vi "5492_AutonomousTurn.vi"(8 "error in (no error)":errorcluster, 9 "RobotDriveDevRef":T1={"DevStatus"={"status"=FALSE, "code"=0, "source"=""}, "Motors[]"=[], "Square Inputs"=FALSE, "Max Output"=1.0}, 10 "Yaw Goallll":dbl) -> (0 "error out (no error)":errorcluster, 1 "RobotDriveDevRef Output":T1={"DevStatus"={"status"=FALSE, "code"=0, "source"=""}, "Motors[]"=[], "Square Inputs"=FALSE, "Max Output"=1.0})   [LabVIEW 2016]
uses:
  <vilib>/Rock Robotics/WPI/RobotDrive/WPI_RobotDriveDevRef.ctl
  <vilib>/Rock Robotics/WPI/MotorControl/WPI_MotorControlDeviceRef.ctl
  <vilib>/Rock Robotics/WPI/MotorControl/WPI_MotorControlType.ctl
  <vilib>/Rock Robotics/SystemInterfaces/DIO/FPGA_DIOPWMChannel.ctl
  <vilib>/Rock Robotics/WPI/PWM/WPI_PWMDeadband.ctl
  <vilib>/Rock Robotics/WPI/ThirdParty/CanMotor/TalonSRX/WPI_CANTalonSRX_APIControlMode.ctl
  <vilib>/Rock Robotics/WPI/RobotDrive/WPI_RobotDriveSafetyCheck.vi
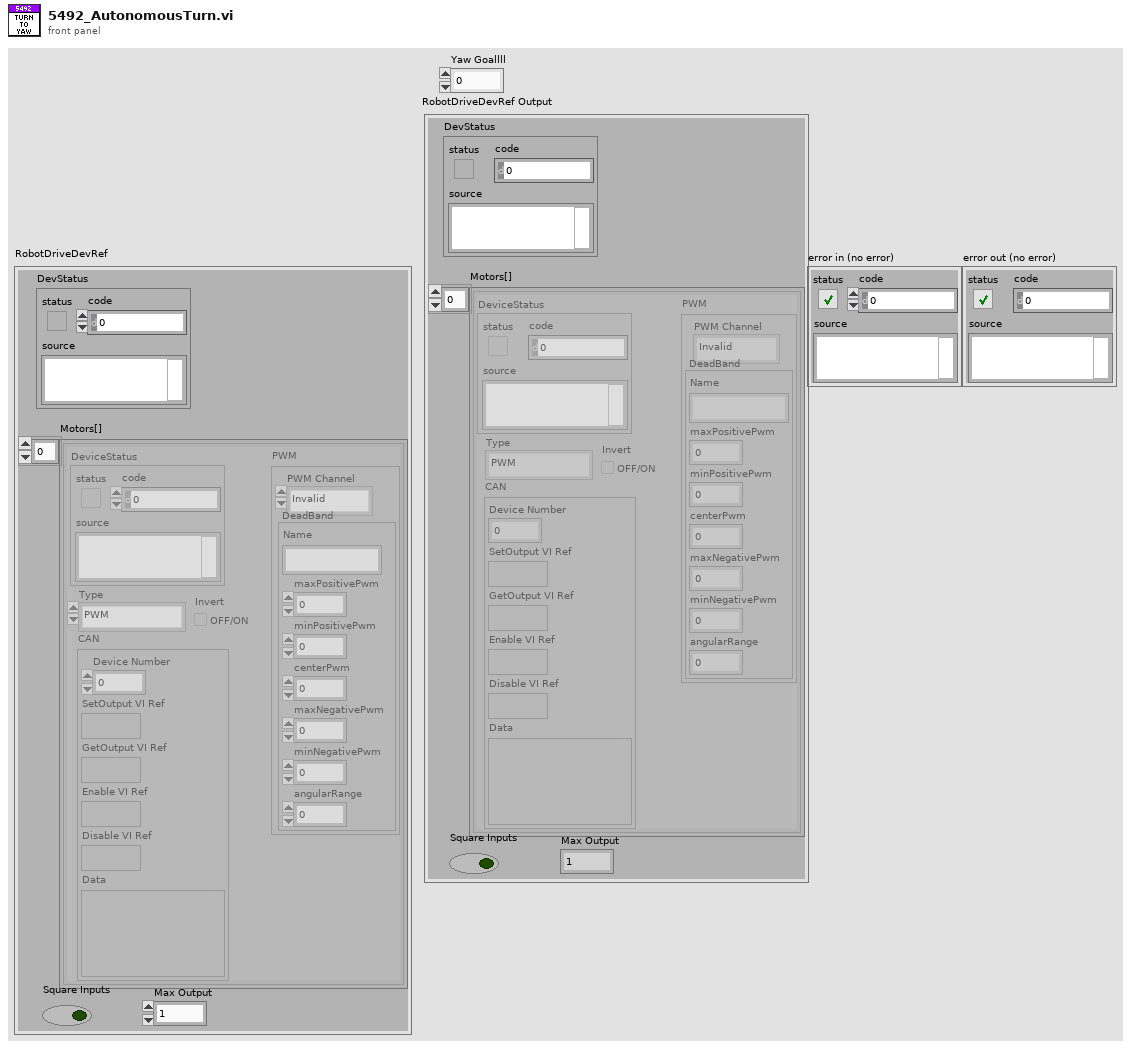
[diagram p1: front panel]
types:
  T1 = typedef "WPI_RobotDriveDevRef.ctl" = cluster{"DevStatus":errorcluster, "Motors[]":T2[], "Square Inputs":bool, "Max Output":dbl}
  T2 = typedef "WPI_MotorControlDeviceRef.ctl" = cluster{"DeviceStatus":errorcluster, "Type":T3, "PWM":cluster{"PWM Channel":T4, "DeadBand":T5}, "CAN":cluster{"Device Number":u8, "SetOutput VI Ref":variant, "GetOutput VI Ref":variant, "Enable VI Ref":variant, "Disable VI Ref":variant, "Data":variant}, "Invert":bool}
  T3 = typedef "WPI_MotorControlType.ctl" = enum16{"PWM", "CAN"}
  T4 = typedef "FPGA_DIOPWMChannel.ctl" = enum8{"PWM 0", "PWM 1", "PWM 2", "PWM 3", "PWM 4", "PWM 5", "PWM 6", "PWM 7", "PWM 8", "PWM 9", "PWM MXP 0", "PWM MXP 1", "PWM MXP 2", "PWM MXP 3", "PWM MXP 4", "PWM MXP 5", "PWM MXP 6", "PWM MXP 7", "PWM MXP 8", "PWM MXP 9", "Invalid"}
  T5 = typedef "WPI_PWMDeadband.ctl" = cluster{"Name":string, "maxPositivePwm":i32, "minPositivePwm":i32, "centerPwm":i32, "maxNegativePwm":i32, "minNegativePwm":i32, "angularRange":u16}
  T6 = typedef "WPI_CANTalonSRX_APIControlMode.ctl" = enum8{"Percent VBus", "Speed", "Position", "Slave", "Unchanged / Invalid", "Voltage Compensation", "Current", "Motion Profile", "Motion Magic"}
  T7 = cluster{"Yaw":dbl, "Roll":dbl, "Pitch":dbl, "Heading":dbl, "Fused Heading":dbl}
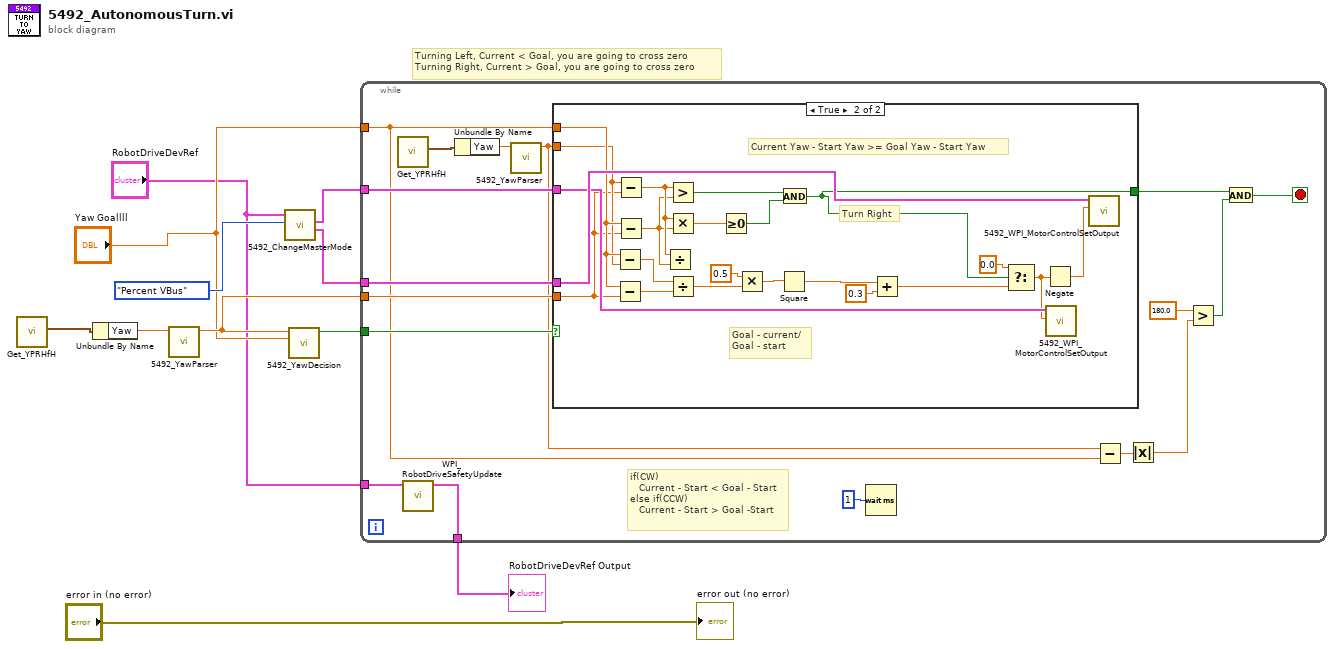
[diagram p0: block diagram]
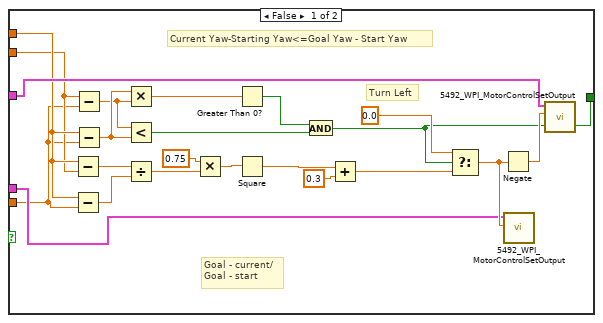
[diagram p2: hidden frame]
diagram:
  # "Turning Left, Current < Goal, you are going to cross zero\nTurning Right, Current > Goal, you are going to cross zero"
  n1 = call <vilib>:"Get_YPRHfH.vi"() -> ("YRPHfH"=w4:T7)  [unwired: 11 in]
  n2 = Unbundle By Name(w4) -> ("Yaw"=w8:dbl)
  n3 = call "5492_YawParser.vi"("Yaw"=w8) -> ("Parsed Yaw"=w6:dbl)  [unwired: 10 in]
  n4 = call "5492_ChangeMasterMode.vi"("Control Mode"=WPI_CANTalonSRX_APIControlMode."Percent VBus", "RobotDriveDevRef"="RobotDriveDevRef") -> ("CAN Talon SRX Right"=w9:T2, "CAN Talon SRX Ref Left"=w10:T2)  [unwired: 7 in, 1 out]
  n5 = call "5492_YawDecision.vi"("Yaw Goallll"="Yaw Goallll", "Parsed Yaw"=w6) -> ("Right???"=w7:bool)  [unwired: 9 in]
  n6 = while {
    tunnel: w10 -> [w27]
    tunnel: w9 -> [w26]
    tunnel: w7 -> [w25]
    tunnel: w6 -> [w23]
    tunnel: "Yaw Goallll" -> [w20]
    tunnel: "RobotDriveDevRef" -> [w13]
    tunnel: [w12] -> w1
    stop <- w14 stop-if-true
    # "if(CW)\n   Current - Start < Goal - Start\nelse if(CCW)\n   Current - Start > Goal -Start"
    n7 = call <vilib>:"Get_YPRHfH.vi"() -> ("YRPHfH"=w22:T7)  [unwired: 11 in]
    n8 = call <vilib>:"WPI_RobotDriveSafetyUpdate.vi"("RobotDriveDevRef"=w13) -> ("RobotDriveDevRef"=w12:T1)  [unwired: 1 in, 9 out]
    n9 = Unbundle By Name(w22) -> ("Yaw"=w24:dbl)
    n10 = call "5492_YawParser.vi"("Yaw"=w24) -> ("Parsed Yaw"=w21:dbl)  [unwired: 10 in]
    n11 = case shown="True" w25 {
      tunnel: w27 -> [w50 w70]
      tunnel: w26 -> [w44 w71]
      tunnel: w21 -> [w31 w54]
      tunnel: w23 -> [w30 w53]
      tunnel: w20 -> [w32 w61]
      tunnel: [w46 w66] -> w15
      frame False {
        # "Current Yaw-Starting Yaw<=Goal Yaw - Start Yaw"
        # "Goal - current/\nGoal - start"
        # "Turn Left"
        n12 = Subtract(x=w32, y=w31) -> (x-y=w33:dbl)
        n13 = Subtract(x=w32, y=w30) -> (x-y=w34:dbl)
        n14 = Subtract(x=w31, y=w30) -> (x-y=w42:dbl)
        n15 = Subtract(x=w32, y=w30) -> (x-y=w43:dbl)
        n16 = Multiply(x=w43, y=w42) -> (x*y=w41:dbl)
        n17 = Less?(x=w42, y=w43) -> (x < y?=w45:bool)
        n18 = Divide(x=w33, y=w34) -> (x/y=w37:dbl)
        n19 = Multiply(x=0.75, y=w37) -> (x*y=w36:dbl)
        n20 = Greater Than 0?(x=w41) -> (x > 0?=w40:bool)
        n21 = Square(x=w36) -> (x^2=w35:dbl)
        n22 = And(x=w40, y=w45) -> (x .and. y?=w46:bool)
        n23 = Add(x=w35, y=0.3) -> (x+y=w29:dbl)
        n24 = Select(t=0.0, s=w46, f=w29) -> (s? t:f=w48:dbl)
        n25 = Negate(x=w48) -> (-x=w49:dbl)
        n26 = call "5492_WPI_MotorControlSetOutput.vi"("Output"=w48, "MotorControlDevRef"=w44) -> ()  [unwired: 7 in, 3 out]
        n27 = call "5492_WPI_MotorControlSetOutput.vi"("Output"=w49, "MotorControlDevRef"=w50) -> ()  [unwired: 7 in, 3 out]
      }
      frame True {
        # "Current Yaw - Start Yaw >= Goal Yaw - Start Yaw"
        # "Goal - current/\nGoal - start"
        # "Turn Right"
        n28 = Subtract(x=w61, y=w54) -> (x-y=w60:dbl)
        n29 = Subtract(x=w61, y=w53) -> (x-y=w59:dbl)
        n30 = Subtract(x=w54, y=w53) -> (x-y=w63:dbl)
        n31 = Subtract(x=w61, y=w53) -> (x-y=w62:dbl)
        n32 = Divide(x=w63, y=w62) -> ()  [unwired: 1 out]
        n33 = Greater?(x=w63, y=w62) -> (0:w67:bool)
        n34 = Multiply(x=w63, y=w62) -> (x*y=w65:dbl)
        n35 = Divide(x=w60, y=w59) -> (x/y=w56:dbl)
        n36 = Greater Or Equal To 0?(x=w65) -> (x >= 0?=w64:bool)
        n37 = Multiply(x=0.5, y=w56) -> (x*y=w57:dbl)
        n38 = Square(x=w57) -> (x^2=w58:dbl)
        n39 = And(x=w67, y=w64) -> (x .and. y?=w66:bool)
        n40 = Add(x=w58, y=0.3) -> (x+y=w51:dbl)
        n41 = Select(t=0.0, s=w66, f=w51) -> (s? t:f=w68:dbl)
        n42 = Negate(x=w68) -> (-x=w69:dbl)
        n43 = call "5492_WPI_MotorControlSetOutput.vi"("Output"=w68, "MotorControlDevRef"=w70) -> ()  [unwired: 7 in, 3 out]
        n44 = call "5492_WPI_MotorControlSetOutput.vi"("Output"=w69, "MotorControlDevRef"=w71) -> ()  [unwired: 7 in, 3 out]
      }
    }
    n45 = Wait (ms)(milliseconds to wait=u32 1) -> ()  [unwired: 1 out]
    n46 = Subtract(x=w21, y=w20) -> (x-y=w19:dbl)
    n47 = Absolute Value(x=w19) -> (abs(x)=w18:dbl)
    n48 = Greater?(x=180.0, y=w18) -> (0:w16:bool)
    n49 = And(x=w15, y=w16) -> (x .and. y?=w14:bool)
  }
  "RobotDriveDevRef Output" <- w1
  "error out (no error)" <- "error in (no error)"
